vi "pulseshaping.vi"(9 "数组":cdb[](array[numeric]), 11 "簇":T1 {"簇"."pulse shaping filter" items=["none", "Raised Cosine", "Root Raised Cos", "Gsussian"]; "簇"."modulation type" items=["FSK", "PSK", "QAM", "MSK", "PAM", "ASK"]}) -> (3 "output":cdb[](array[numeric]) caption="X * Y")   [LabVIEW 2013]
uses:
  <vilib>/addons/Modulation/niDMT.lvlib
  <vilib>/Analysis/NI_AALPro.lvlib
  <vilib>/Analysis/2dsp.llb/Upsample (CDB).vi
  <vilib>/Analysis/2dsp.llb/1D Convolution (CDB).vi
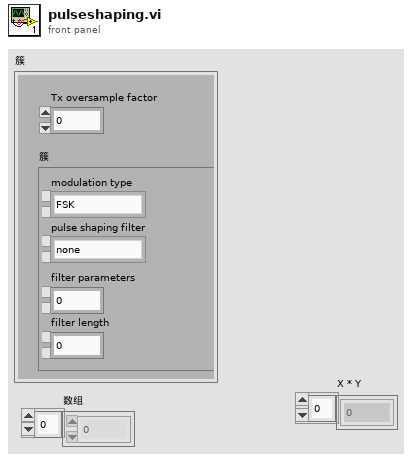
[diagram p1: front panel]
types:
  T1 = cluster{"Tx oversample factor":i32, "簇":cluster{"modulation type":u16, "pulse shaping filter":u16, "filter parameters":dbl, "filter length":i32}}
  T2 = cluster{"modulation type":u16, "pulse shaping filter":u16, "filter parameters":dbl, "filter length":i32}
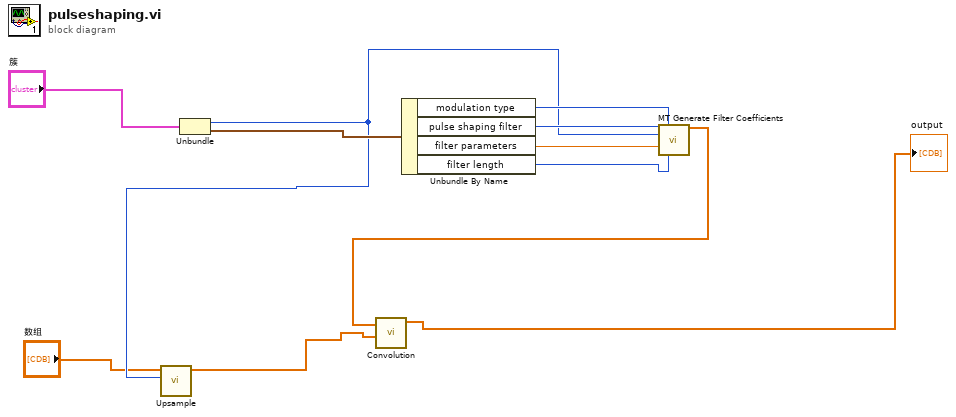
[diagram p0: block diagram]
diagram:
  n1 = Unbundle("簇") -> ("Tx oversample factor"=w2:i32, "簇"=w3:T2)
  n2 = call-poly <vilib>:"Upsample.vi"("upsampling factor"=w2, "X"="数组") -> ("Upsampled Array"=w6:cdb[])  [unwired: 8 in, 1 out]
  n3 = Unbundle By Name(w3) -> ("modulation type"=w10:u16, "pulse shaping filter"=w11:u16, "filter parameters"=w8:dbl, "filter length"=w9:i32)
  n4 = call <vilib>:"MT Generate Filter Coefficients.vi"("pulse shaping filter (none)"=w11, "modulation type"=w10, "pulse shaping samples per symbol (16)"=w2, "filter parameter"=w8, "filter length (symbols)"=w9) -> ("pulse shaping filter coefficients"=w7:dbl[])  [unwired: 8 in, 2 out]
  n5 = call-poly <vilib>:"Convolution.vi"("Y"=w6, "X"=w7) -> ("X * Y"=→"output":cdb[])  [unwired: 8 in, 1 out]
